vi "Test Panel - Data Save (SubVI).vi"(8 "error in":errorcluster) -> (0 "error Out":errorcluster, 2 "Cancel?":bool, 3 "Select Report Path out":path)   [LabVIEW 2019]
uses:
  Controls/Add test-state.ctl
  Controls/eFGV States.ctl
panel:
  in  "Test Name":path
  in  "OK":bool
  in  "Cancel":bool
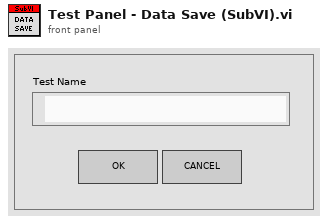
[diagram p1: front panel]
types:
  T1 = typedef "Add test-state.ctl" = enum16{"Init", "Idle", "Add", "Load Station", "Load", "Check Device", "Close", "Exit"}
  T2 = typedef "eFGV States.ctl" = enum16{"Init", "Read", "Write", "Exit"}
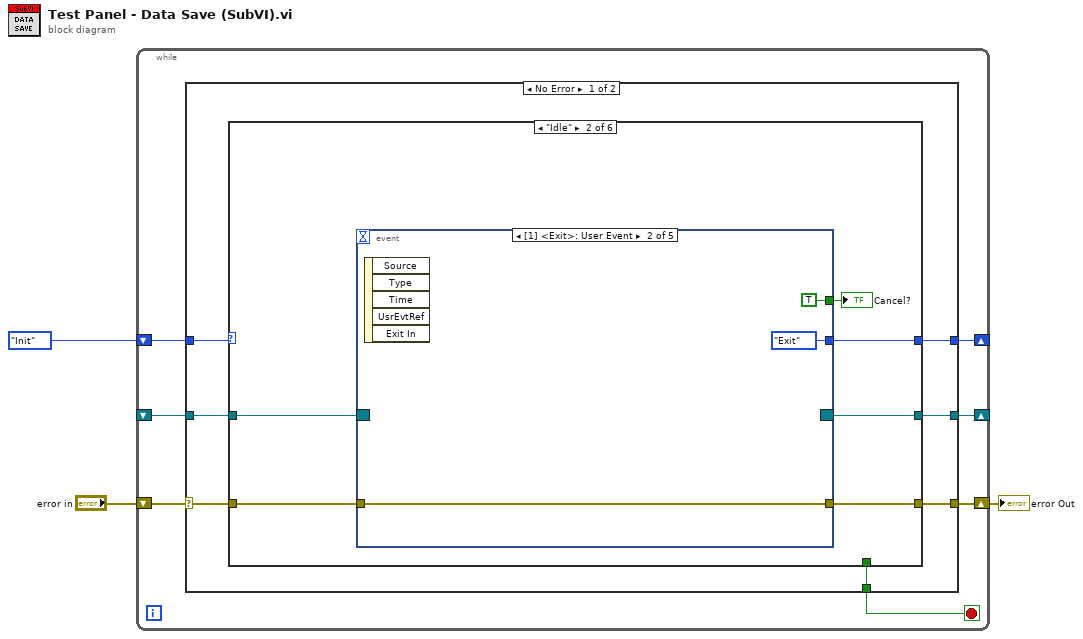
[diagram p0: block diagram]
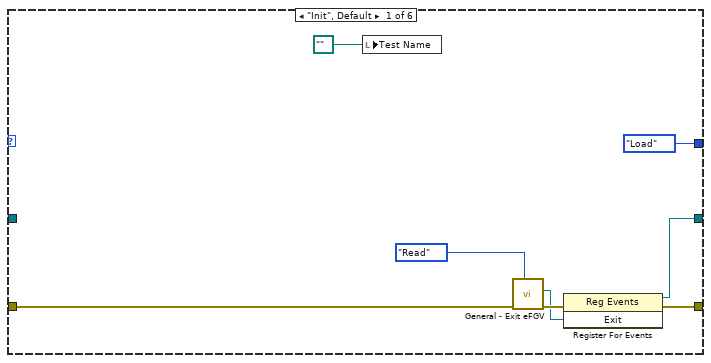
[diagram p2: hidden frame]
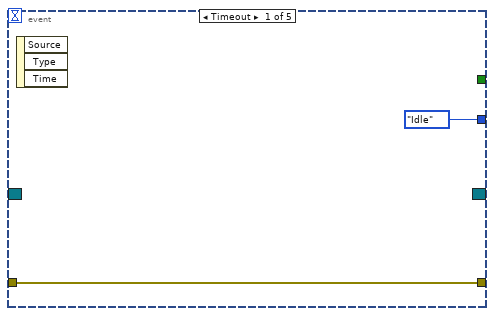
[diagram p3: hidden frame]
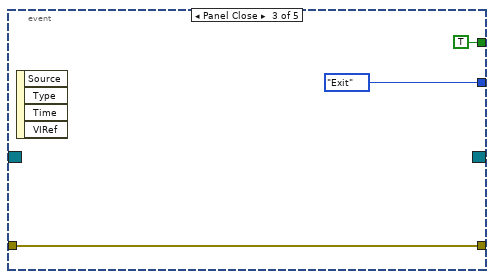
[diagram p4: hidden frame]
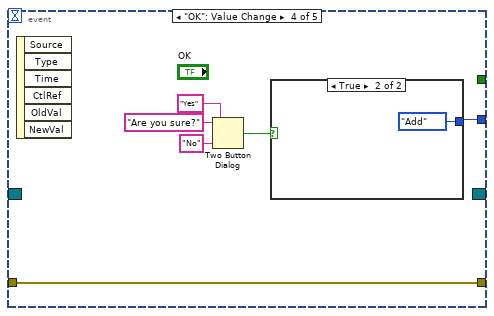
[diagram p5: hidden frame]
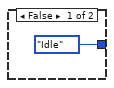
[diagram p6: hidden frame]
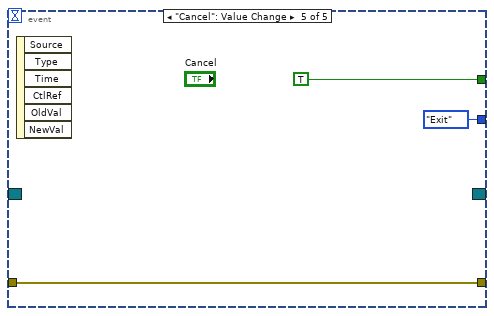
[diagram p7: hidden frame]
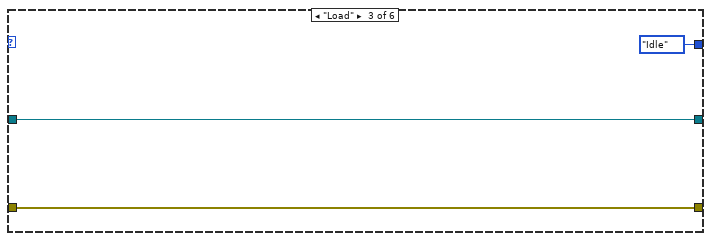
[diagram p8: hidden frame]
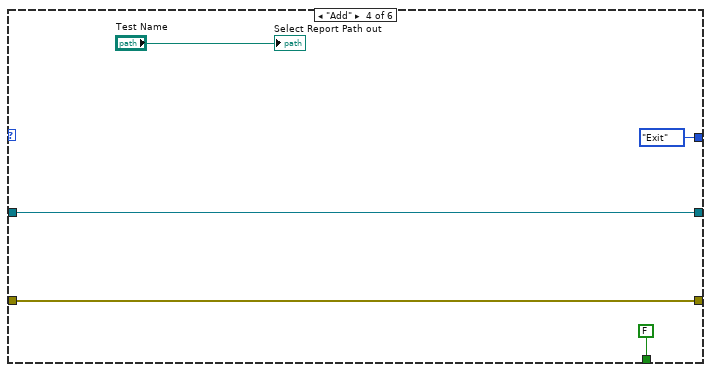
[diagram p9: hidden frame]
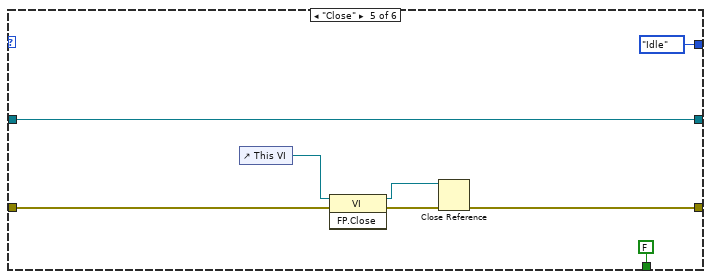
[diagram p10: hidden frame]
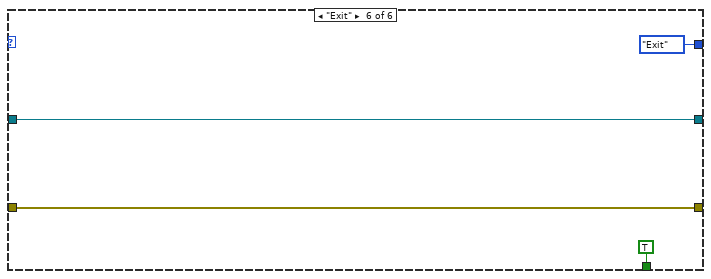
[diagram p11: hidden frame]
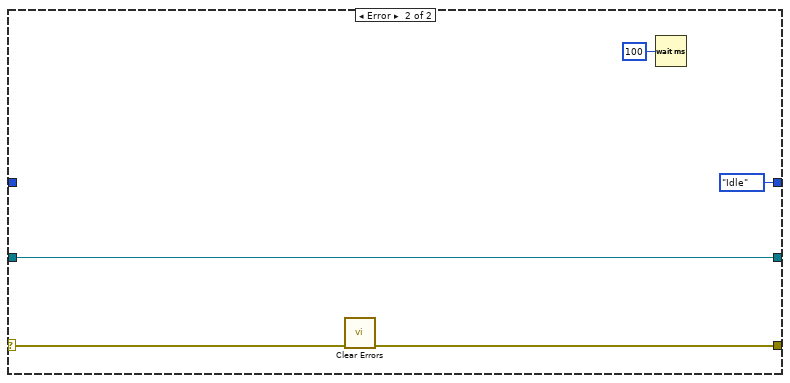
[diagram p12: hidden frame]
diagram:
  n1 = while {
    shift-right: [w9] -> w1
    shift-left: "error in" -> [w10]
    shift-right: [w7] -> _
    shift-left: Add_test-state."Init" -> [w8]
    shift-right: [w5] -> _
    shift-left: _ -> [w4]
    stop <- w6 stop-if-true
    n2 = case shown="No Error" w10 {
      selector: w10 -> [w17 w75]
      tunnel: [w16 w73] -> w9
      tunnel: w8 -> [w15 _]
      tunnel: [w14 Add_test-state."Idle"] -> w7
      tunnel: [w13 _] -> w6
      tunnel: [w12 w74] -> w5
      tunnel: w4 -> [w11 w74]
      frame No Error {
        n3 = case shown="\"Idle\"" w15 {
          tunnel: w17 -> [w20 w31 w51 w55 w62 w70]
          tunnel: [w23 w30 w51 w55 w60 w70] -> w16
          tunnel: [Add_test-state."Load" w29 Add_test-state."Idle" Add_test-state."Exit" Add_test-state."Idle" Add_test-state."Exit"] -> w14
          tunnel: [_ _ _ FALSE FALSE TRUE] -> w13
          tunnel: [w21 w27 w53 w56 w66 w69] -> w12
          tunnel: w11 -> [_ w28 w53 w56 w66 w69]
          frame "Init", Default {
            n4 = local write "Test Name"(path "" ("Select Report Path")) -> ()
            n5 = call "General - Exit eFGV.vi"("eFGV States"=eFGV_States."Read", "error in (no error)"=w20) -> ("error out"=w24:errorcluster, "Exit"=w22:refnum<user-event>)  [unwired: 7 in, 1 out]
            n6 = register-events(error in=w24, w22) -> (reference out=w21:refnum<event-registration>, error out=w23:errorcluster)  [unwired: 1 in]
          }
          frame "Idle" {
            n7 = event shown="[1] <Exit>: User Event" {
              selector: w28 -> [_ _ _ _ _]
              dyn-events: [_ _ _ _ _] -> w27
              timeout: _ -> [_ _ _ _ _]
              tunnel: w31 -> [w33 w36 w39 w45 w49]
              tunnel: [w33 w36 w39 w45 w49] -> w30
              tunnel: [Add_test-state."Idle" Add_test-state."Exit" Add_test-state."Exit" w40 Add_test-state."Exit"] -> w29
              tunnel: [_ TRUE TRUE _ TRUE] -> w26
              event Timeout {
                n8 = event-data() -> ()  [unwired: 1 in, 3 out]
              }
              event User Event {
                n9 = event-data() -> ()  [unwired: 1 in, 5 out]
              }
              event Panel Close {
                n10 = event-data() -> ()  [unwired: 1 in, 4 out]
              }
              event "OK": Value Change {
                n11 = event-data() -> ()  [unwired: 1 in, 6 out]
                n12 = Two Button Dialog(message="Are you sure?", 1:"No" ("F button name (\"Cancel\")"), 2:"Yes" ("T button name (\"OK\")")) -> (T button?=w41:bool)
                n13 = case shown="True" w41 {
                  tunnel: [Add_test-state."Idle" Add_test-state."Add"] -> w40
                  frame False {
                  }
                  frame True {
                  }
                }
              }
              event "Cancel": Value Change {
                n14 = event-data() -> ()  [unwired: 1 in, 6 out]
              }
            }
            "Cancel?" <- w26
          }
          frame "Load" {
          }
          frame "Add" {
            "Select Report Path out" <- "Test Name"
          }
          frame "Close" {
            n15 = control-ref of="This VI"() -> (w61:refnum<vi>)
            n16 = invoke class="VI" method="FP.Close"(reference=w61, error in=w62) -> (reference out=w59:refnum<vi>, error out=w63:errorcluster)  [unwired: 1 in, 1 out]
            n17 = Close Reference(reference=w59, error in (no error)=w63) -> (error out=w60:errorcluster)
          }
          frame "Exit" {
          }
        }
      }
      frame Error {
        n18 = call <vilib>:"Clear Errors.vi"("error in (no error)"=w75) -> ("error out"=w73:errorcluster)  [unwired: 5 in, 1 out]
        n19 = Wait (ms)(milliseconds to wait=u32 100) -> ()  [unwired: 1 out]
      }
    }
  }
  "error Out" <- w1
